vi "揭晓游戏结局.vi"(1 "地图":i32[][](array[numeric])) -> (0 "输出地图":i32[][](array[numeric]))   [LabVIEW 2017]
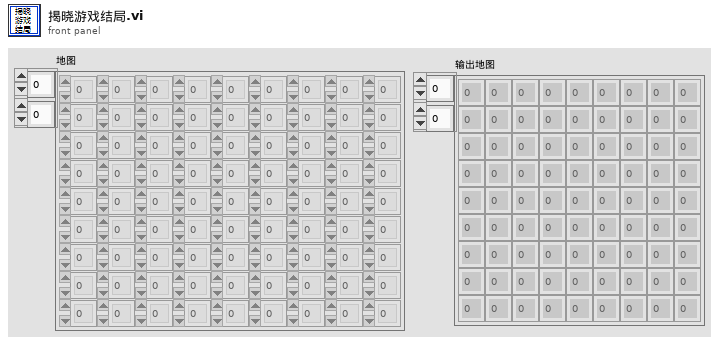
[diagram p1: front panel]
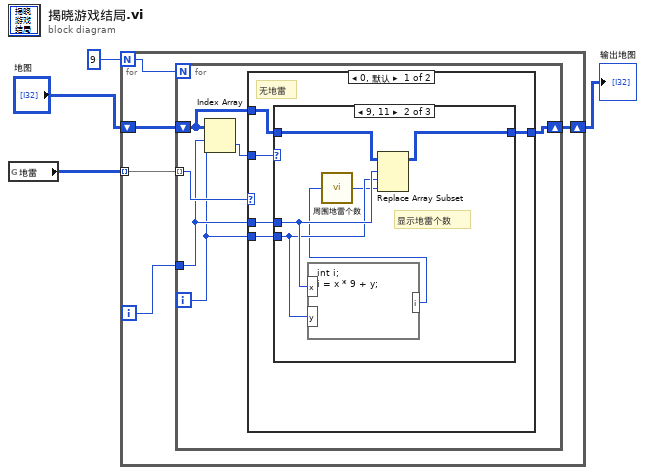
[diagram p0: block diagram]
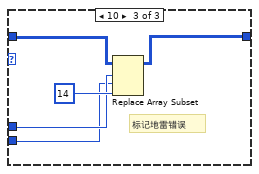
[diagram p3: hidden frame]
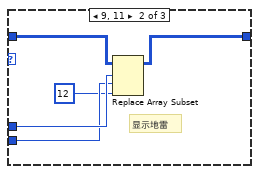
[diagram p5: hidden frame]
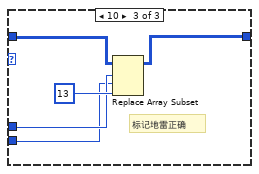
[diagram p6: hidden frame]
diagram:
  n1 = global read "全局 地雷数组.vi" "地雷"() -> (w1:i16[][])
  n2 = for {
    N: 9 -> [w7]
    shift-right: [w8] -> w4
    shift-left: "地图" -> [w9]
    tunnel: w1 -> [w5] mode=indexing
    i -> [w6]
    n3 = for {
      N: w7 -> [_]
      shift-right: [w12] -> w8
      shift-left: w9 -> [w13]
      tunnel: w6 -> [w11]
      tunnel: w5 -> [w14] mode=indexing
      i -> [w10]
      n4 = Index Array(array=w13, index (row)=w11, index (col)=w10) -> (element=w15:i32)
      n5 = case shown="0, 默认" w14 {
        tunnel: w15 -> [w18 w37]
        tunnel: w13 -> [w19 w36]
        tunnel: [w20 w35] -> w12
        tunnel: w11 -> [w17 w34]
        tunnel: w10 -> [w16 w33]
        frame 0, Default {
          # "无地雷"
          n6 = case shown="9, 11" w18 {
            tunnel: w19 -> [w21 w27 w31]
            tunnel: [w21 w26 w28] -> w20
            tunnel: w17 -> [_ w25 w30]
            tunnel: w16 -> [_ w24 w29]
            frame 0..8, Default {
              # "无地雷"
            }
            frame 9, 11 {
              # "显示地雷个数"
              n7 = formula code="int i;\ni = x * 9 + y;"("x"=w25, "y"=w24) -> ("i"=w23:i32)
              n8 = call "周围地雷个数.vi"("索引"=w23) -> ("数值"=w22:i32)
              n9 = Replace Array Subset(array=w27, new element=w22, index (row)=w25, index (col)=w24) -> (w26:i32[][])
            }
            frame 10 {
              # "标记地雷错误"
              n10 = Replace Array Subset(array=w31, new element=14, index (row)=w30, index (col)=w29) -> (w28:i32[][])
            }
          }
        }
        frame 1 {
          # "有地雷"
          n11 = case shown="0..8, 默认" w37 {
            tunnel: w36 -> [w38 w43 w47]
            tunnel: [w38 w42 w44] -> w35
            tunnel: w34 -> [_ w41 w46]
            tunnel: w33 -> [_ w40 w45]
            frame 0..8, Default {
              # "有地雷，不可能的情况"
            }
            frame 9, 11 {
              # "显示地雷"
              n12 = Replace Array Subset(array=w43, new element=12, index (row)=w41, index (col)=w40) -> (w42:i32[][])
            }
            frame 10 {
              # "标记地雷正确"
              n13 = Replace Array Subset(array=w47, new element=13, index (row)=w46, index (col)=w45) -> (w44:i32[][])
            }
          }
        }
      }
    }
  }
  "输出地图" <- w4
